vi "DataView.vi"() -> ()   [LabVIEW 2020]
uses:
  <vilib>/Native 3D Graph/xcontrol/3DPC_SurfacePlot.xctl
panel:
  in  "Filename":string
  in  "File DIrectory path":path
  in  "Y Step Size":dbl format="%#_13g"
  in  "X Step Size":dbl format="%#_13g"
  in  "Line Count":i32
  in  "Pixel Count":i32
  out "Surface Plot":refnum<class "Base Datatype.lvclass">[](xcontrol)
  in  "Reset Img":bool
  in  "Save Img":bool
  in  "Select View Mode":enum32{"Max Amp", "Layer View"}(radio)
  in  "Layer Number":dbl
  out "File Open Success":bool
  in  "H5 Path":path
  in  "Open File":bool
  in  "Colormap Selector":T1(ring)=enum."gray"
  out "Image Display":i32[][](graph)
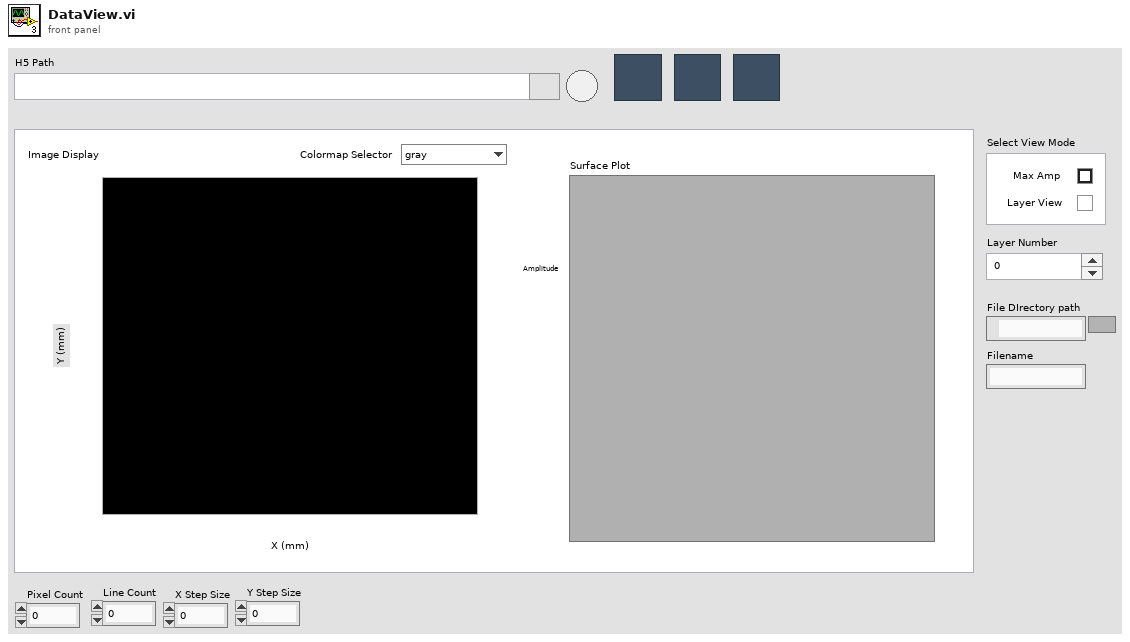
[diagram p1: front panel]
types:
  T1 = enum16{"fire", "rainbow", "gray", "inverse gray", "ice", "original"}
  T2 = typedef "imagedata.ctl" = cluster{"image type":i32, "image depth":i32, "image":u8[], "mask":u8[], "colors":u32[], "Rectangle":cluster{"left":i16, "top":i16, "right":i16, "bottom":i16}}
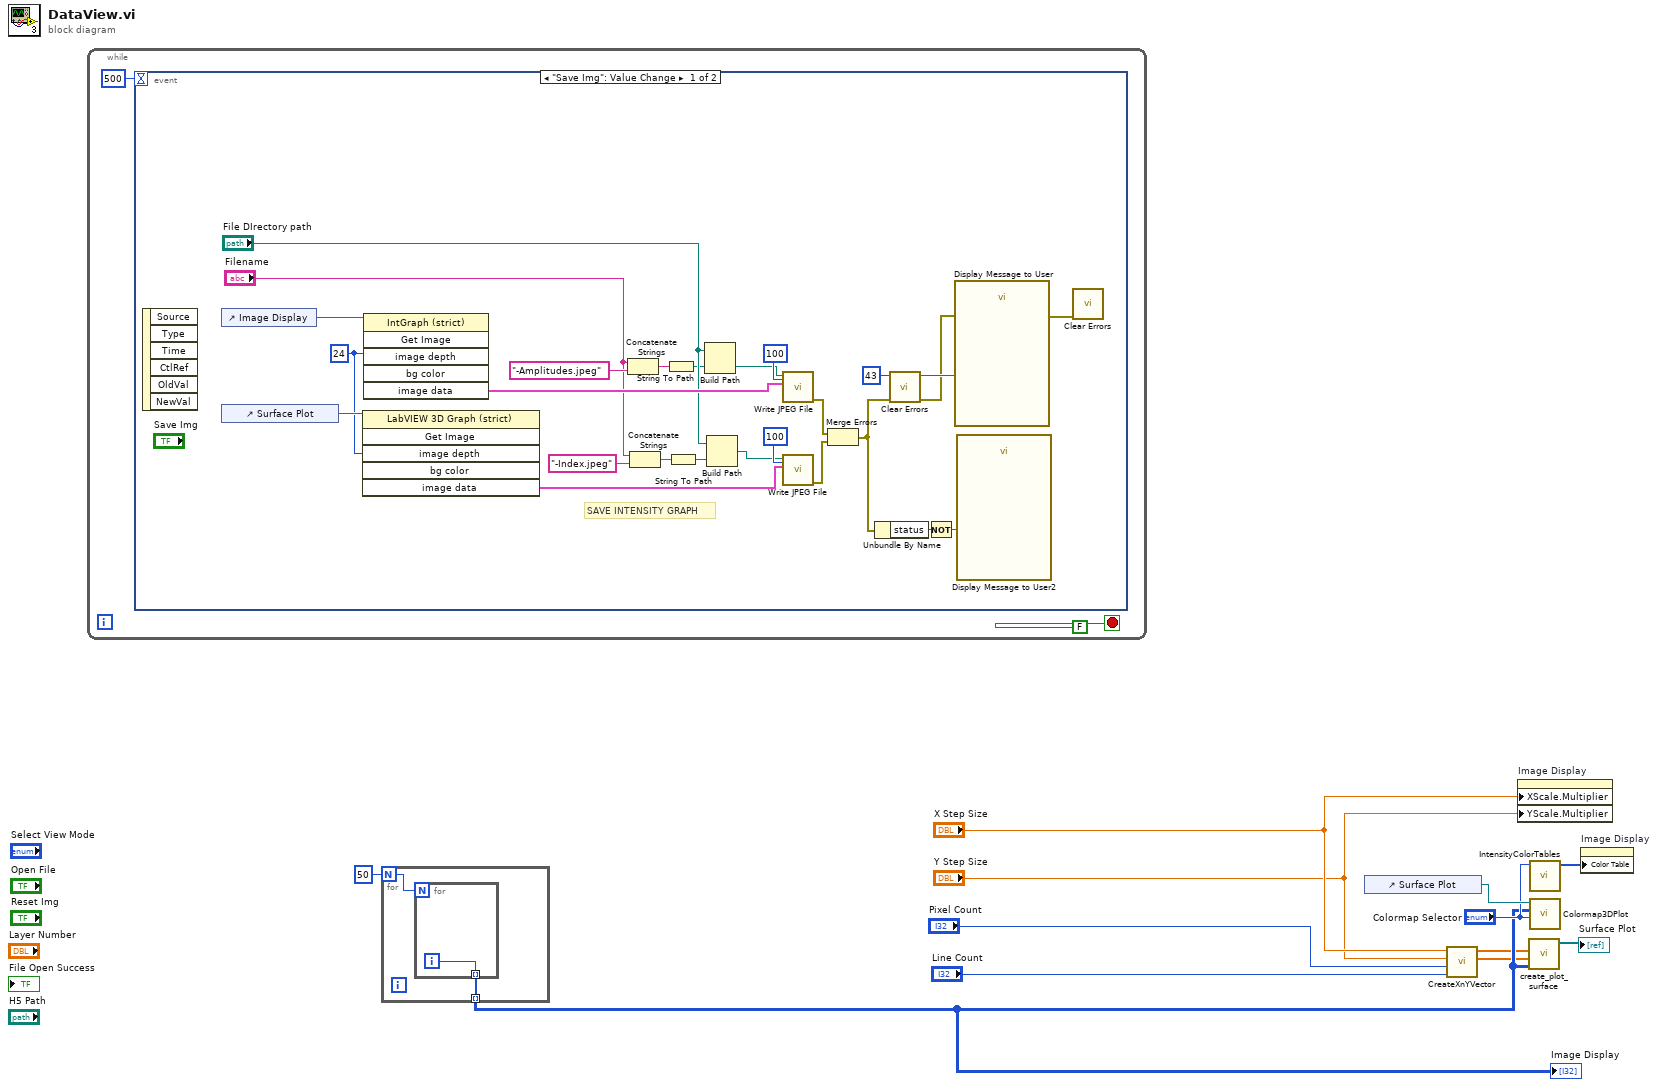
[diagram p0: block diagram]
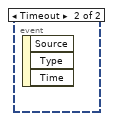
[diagram p2: hidden frame]
diagram:
  n1 = while {
    stop <- FALSE stop-if-true
    n2 = event shown="[0] \"Save Img\": Value Change" {
      selector: _ -> [_ _]
      dyn-events: _ -> [_ _]
      timeout: 500 -> [_ _]
      event "Save Img": Value Change {
        w15 = 24
        # "SAVE INTENSITY GRAPH"
        n3 = event-data() -> ()  [unwired: 1 in, 6 out]
        n4 = control-ref of="Image Display"() -> (w38:refnum<vi>)
        n5 = control-ref of="Surface Plot"() -> (w32:refnum<vi>)
        n6 = invoke class="LabVIEW 3D Graph (strict)" method="Get Image"(reference=w32, "image depth"=w15) -> ("image data"=w30:T2)  [unwired: 4 in, 5 out]
        n7 = invoke class="IntGraph (strict)" method="Get Image"(reference=w38, "image depth"=w15) -> ("image data"=w39:T2)  [unwired: 4 in, 5 out]
        n8 = Concatenate Strings("Filename", "-Amplitudes.jpeg" ("string")) -> (w24:string)
        n9 = Concatenate Strings("Filename", "-Index.jpeg" ("string")) -> (w21:string)
        n10 = String To Path(string=w24) -> (path=w25:path)
        n11 = String To Path(string=w21) -> (path=w20:path)
        n12 = Build Path(base path="File DIrectory path", name or relative path=w25) -> (appended path=w27:path)
        n13 = Build Path(base path="File DIrectory path", name or relative path=w20) -> (appended path=w28:path)
        n14 = call <vilib>:"Write JPEG File.vi"("quality (80)"=100, "image data"=w39, "path to JPEG file"=w27) -> ("error out"=w36:errorcluster)  [unwired: 7 in, 1 out]
        n15 = call <vilib>:"Write JPEG File.vi"("quality (80)"=100, "image data"=w30, "path to JPEG file"=w28) -> ("error out"=w29:errorcluster)  [unwired: 7 in, 1 out]
        n16 = Merge Errors(w36, w29) -> (w17:errorcluster)
        n17 = Unbundle By Name(w17) -> ("status"=w18:bool)
        n18 = call <vilib>:"Clear Errors.vi"("error in (no error)"=w17, "specific error code to clear (0: all)"=43) -> ("error out"=w34:errorcluster, "specific error cleared?"=w35:bool)  [unwired: 4 in]
        n19 = Not(x=w18) -> (.not. x?=w16:bool)
        n20 = call "Display Message to User"("error in (no error)"=w34, "Enable"=w35) -> ("error out"=w33:errorcluster)  [unwired: 8 in, 1 out]
        n21 = call "Display Message to User2"("Enable"=w16) -> ()  [unwired: 9 in, 2 out]
        n22 = call <vilib>:"Clear Errors.vi"("error in (no error)"=w33) -> ()  [unwired: 5 in, 2 out]
      }
      event Timeout {
        n23 = event-data() -> ()  [unwired: 1 in, 3 out]
      }
    }
  }
  n24 = for {
    N: 50 -> [w42]
    tunnel: [w41] -> w7 mode=indexing
    n25 = for {
      N: w42 -> [_]
      tunnel: [w43] -> w41 mode=indexing
      i -> [w43]
    }
  }
  "Image Display" <- w7
  n26 = control-ref of="Surface Plot"() -> (w10:refnum<vi>)
  n27 = call "CreateXnYVector.vi"("Line Count"="Line Count", "Pixel Count"="Pixel Count", "Y Step Size"="Y Step Size", "X Step Size"="X Step Size") -> ("Array 2"=w5:dbl[], "Array"=w3:dbl[])  [unwired: 6 in]
  n28 = property on="Image Display" class="IntGraph (strict)"("XScale.Multiplier"="X Step Size", "YScale.Multiplier"="Y Step Size") -> ()  [unwired: 2 in, 2 out]
  n29 = call <vilib>:"create_plot_surface.vi"("z matrix"=w7, "y vector"=w5, "x vector"=w3) -> ("plots out"=→"Surface Plot":refnum<class "Base Datatype.lvclass">[])  [unwired: 3 in, 5 out]
  n30 = call "IntensityColorTables.vi"("Map Selector"="Colormap Selector") -> ("Color Map Array"=w8:u32[])  [unwired: 10 in]
  n31 = call "Colormap3DPlot.vi"("Map Selector"="Colormap Selector", "Array"=w7, "Control in"=w10) -> ()  [unwired: 9 in]
  n32 = property on="Image Display" class="IntGraph (strict)"("Color Table"=w8) -> ()  [unwired: 2 in, 2 out]
